vi "Table, Copy Visible Properties.vi"(4 "error in":errorcluster, 6 "Tbl Refnum Dst":refnum<vi>, 7 "Tbl Refnum Src":refnum<vi>) -> (0 "error out":errorcluster, 2 "Tbl Refnum Dst out":refnum<vi>, 3 "Tbl Refnum Src out":refnum<vi>)   [LabVIEW 2010]
doc: "Copies the visibility properties (index, headers, scrollbars, etc.) of the source table to the destination table."
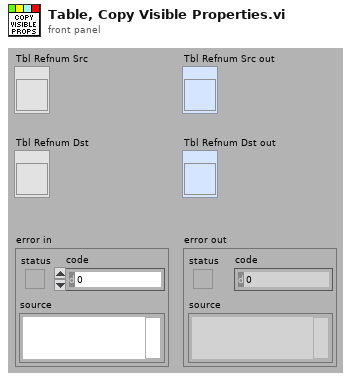
[diagram p1: front panel]
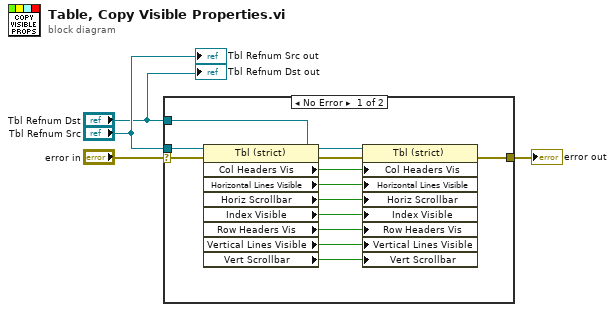
[diagram p0: block diagram]
diagram:
  n1 = case shown="No Error" "error in" {
    selector: "error in" -> [w12 w17]
    tunnel: [w11 w17] -> w4
    tunnel: "Tbl Refnum Dst" -> [w14 _]
    tunnel: "Tbl Refnum Src" -> [w13 _]
    frame No Error {
      n2 = property class="Tbl (strict)"(reference=w13, error in=w12) -> (error out=w15:errorcluster, "Col Headers Vis"=w16:bool, "Horizontal Lines Visible"=w10:bool, "Horiz Scrollbar"=w9:bool, "Index Visible"=w8:bool, "Row Headers Vis"=w7:bool, "Vertical Lines Visible"=w6:bool, "Vert Scrollbar"=w5:bool)  [unwired: 1 out]
      n3 = property class="Tbl (strict)"(reference=w14, error in=w15, "Col Headers Vis"=w16, "Horizontal Lines Visible"=w10, "Horiz Scrollbar"=w9, "Index Visible"=w8, "Row Headers Vis"=w7, "Vertical Lines Visible"=w6, "Vert Scrollbar"=w5) -> (error out=w11:errorcluster)  [unwired: 1 out]
    }
    frame Error {
    }
  }
  "error out" <- w4
  "Tbl Refnum Src out" <- "Tbl Refnum Src"
  "Tbl Refnum Dst out" <- "Tbl Refnum Dst"
